vi "HTVacuum.ProcEvents.vi"(0 "i ref in":refnum<vi>, 5 "error in (no error)":errorcluster) -> (14 "i ref out":refnum<vi>, 19 "error out":errorcluster)   [LabVIEW 2014, in "HTVacuum.lvlib"]
doc: "This method is used to define the events the object will listen to. Add your own events here."
uses:
  HTVacuum.lvlib
  CS_Core/BaseProcess/BaseProcess.event definition.ctl
  CS_Core/CAEObj/CAEObj.event definition.ctl
  CS_Core/BaseProcess/BaseProcess.descriptor string definition.ctl
  CS_Core/BaseProcess/BaseProcess.lvlib
  CS_Core/CAEObj/CAEObj.lvlib
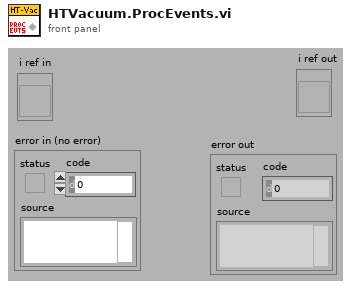
[diagram p1: front panel]
types:
  T1 = typedef "BaseProcess.lvlib/BaseProcess.event definition.ctl" = cluster{"CAEEvtDef":T2, "Data Descriptor":T3}
  T2 = typedef "CAEObj.lvlib/CAEObj.event definition.ctl" = cluster{"URL":string, "enable":bool, "ignoreResID":bool}
  T3 = typedef "BaseProcess.lvlib/BaseProcess.descriptor string definition.ctl" = string
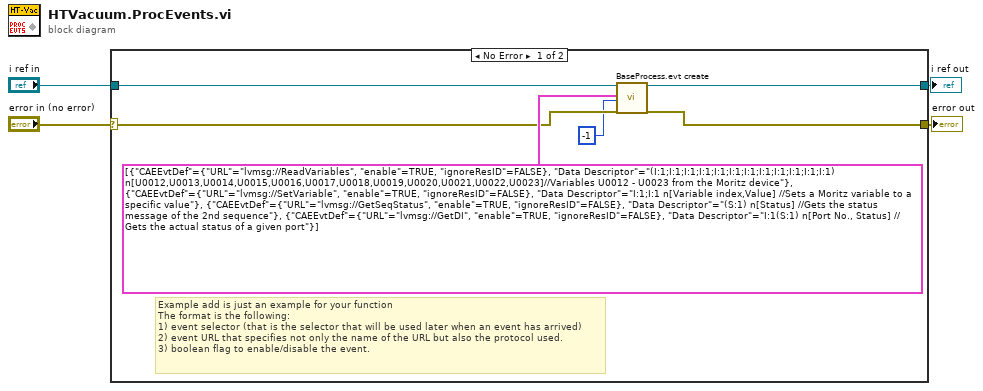
[diagram p0: block diagram]
diagram:
  n1 = case shown="No Error" "error in (no error)" {
    selector: "error in (no error)" -> [w6 w11]
    tunnel: "i ref in" -> [w10 w12]
    tunnel: [w9 w12] -> w3
    tunnel: [w8 w11] -> w2
    frame No Error {
      # "Example add is just an example for your function\nThe format is the following:\n1) event selector (that is the selector that will be used later when an event has arrived)\n2) event URL that specifies not only the name of the URL but also the protocol used.\n3) boolean flag to enable/disable the event."
      n2 = call "BaseProcess.evt create.vi"("i ref in"=w10, "newEvents"=T1[] [{"CAEEvtDef"={"URL"="lvmsg://ReadVariables", "enable"=TRUE, "ignoreResID"=FALSE}, "Data Descriptor"="(I:1;I:1;I:1;I:1;I:1;I:1;I:1;I:1;I:1;I:1;I:1;I:1) n[U0012,U0013,U0014,U0015,U0016,U0017,U0018,U0019,U0020,U0021,U0022,U0023]//Variables U0012 - U0023 from the Moritz device"}, {"CAEEvtDef"={"URL"="lvmsg://SetVariable", "enable"=TRUE, "ignoreResID"=FALSE}, "Data Descriptor"="I:1;I:1 n[Variable index,Value] //Sets a Moritz variable to a specific value"}, {"CAEEvtDef"={"URL"="lvmsg://GetSeqStatus", "enable"=TRUE, "ignoreResID"=FALSE}, "Data Descriptor"="(S:1) n[Status] //Gets the status message of the 2nd sequence"}, {"CAEEvtDef"={"URL"="lvmsg://GetDI", "enable"=TRUE, "ignoreResID"=FALSE}, "Data Descriptor"="I:1(S:1) n[Port No., Status] //Gets the actual status of a given port"}] ("new events"), "ms timeout (10000)"=-1, "error in (no error)"=w6) -> ("i ref out"=w9:refnum<vi>, "error out"=w8:errorcluster)  [unwired: 12 in, 2 out]
    }
    frame Error {
    }
  }
  "i ref out" <- w3
  "error out" <- w2
